vi "ScriptAllIOinCases.vi"(8 "direction":T1, 9 "Case diagrams":refnum<vi>[](array[refnum]), 11 "I/O names":string[](array[string])) -> (3 "IO terminals":refnum<vi>[](array[refnum]))   [LabVIEW 2014]
uses:
  <vilib>/eio/EIO_TerminalDirection.ctl
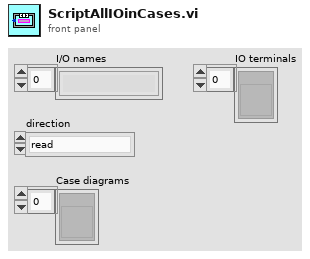
[diagram p1: front panel]
types:
  T1 = typedef "EIO_TerminalDirection.ctl" = enum16{"read", "write", "none", "both"}
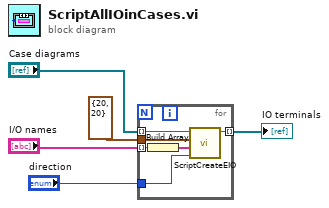
[diagram p0: block diagram]
diagram:
  n1 = for {
    tunnel: [w11] -> w5 mode=indexing
    tunnel: cluster{"Left":i32, "Top":i32} {"Left"=20, "Top"=20} ("Position") -> [w10]
    tunnel: "I/O names" -> [w9] mode=indexing
    tunnel: "direction" -> [w8]
    tunnel: "Case diagrams" -> [w7] mode=indexing
    n2 = Build Array(w9) -> (w6:string[])
    n3 = call "ScriptCreateEIO.vi"("direction"=w8, "nodes links"=w6, "Position"=w10, "TopLevelDiagram in"=w7) -> ("I/O terminal"=w11:refnum<vi>)  [unwired: 4 in, 3 out]
  }
  "IO terminals" <- w5
